vi "finish_photon_stream.vi"(8 "error in (no error)":errorcluster, 11 "picoharp in":refnum<class "picoharp.lvclass">) -> (0 "error out":errorcluster, 3 "picoharp out":refnum<class "picoharp.lvclass">)   [LabVIEW 2015, in "picoharp.lvclass"]
uses:
  picoharp.lvclass
  picoharp.lvclass/picoharp.ctl
  phlib.dll
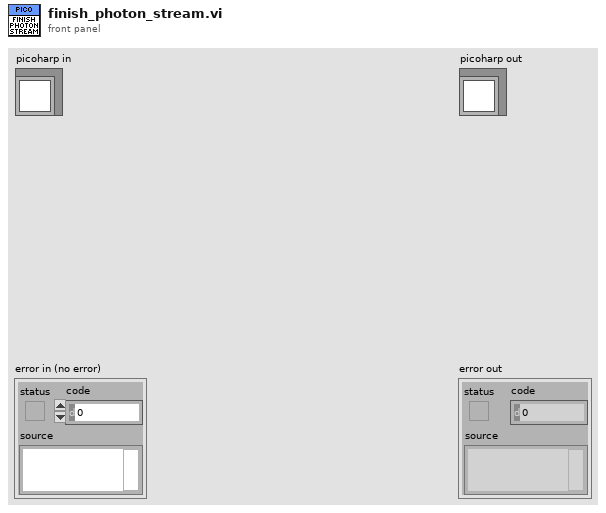
[diagram p1: front panel]
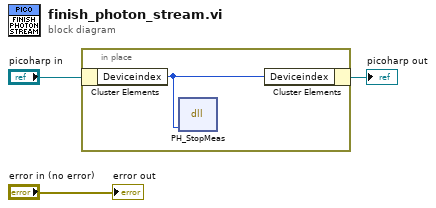
[diagram p0: block diagram]
diagram:
  n1 = in-place {
    n2 = in-place-cluster #1("picoharp in") -> ("Deviceindex"=w4:i32)
    n3 = dll-call lib="phlib.dll" fn="PH_StopMeas" label="pH_StopMeas"("devidx"=w4) -> ()  [unwired: 5 in, 2 out]
    n4 = in-place-cluster #1("Deviceindex"=w4) -> (→"picoharp out":refnum<class "picoharp.lvclass">)
  }
  "error out" <- "error in (no error)"
